vi "Acquire_V2.vi"(5 "Weight Port":refnum<visa-resource-name>, 6 "error in":errorcluster, 7 "GlobalData":T1, 8 "Calibration":variant, 11 "Pressure":refnum<k21>) -> (0 "Weight Port":refnum<visa-resource-name>, 3 "Pressure":refnum<k21>, 4 "error out":errorcluster)   [LabVIEW 2024]
doc: "This the UI responsbile of collection data and display it"
uses:
  controls/GlobalData.ctl
  <vilib>/DAQmx/read.llb/DAQmx Read (Analog 1D DBL NChan 1Samp).vi
  <vilib>/DAQmx/miscellaneous.llb/DAQmx Fill In Error Info.vi
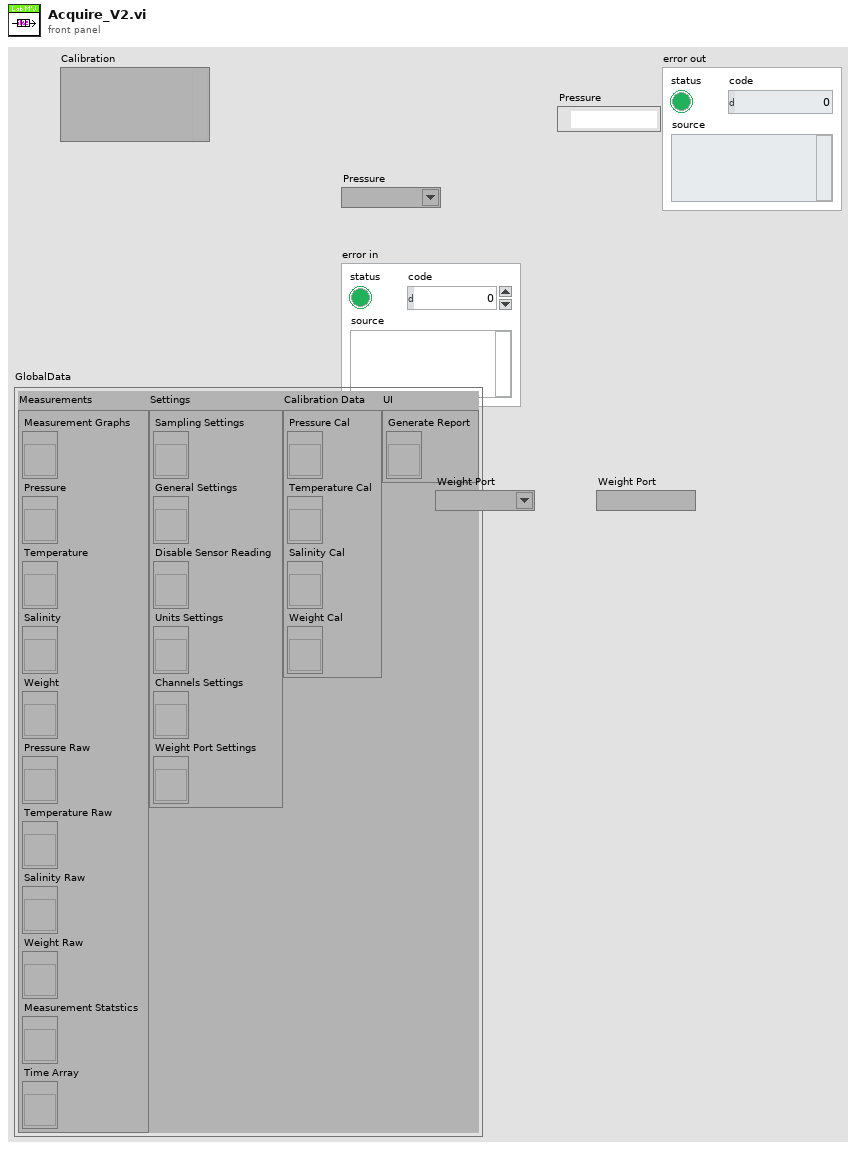
[diagram p1: front panel]
types:
  T1 = typedef "GlobalData.ctl" = cluster{"Measurements":cluster{"Measurement Graphs":refnum<vi>, "Pressure":refnum<vi>, "Temperature":refnum<vi>, "Salinity":refnum<vi>, "Weight":refnum<vi>, "Pressure Raw":refnum<vi>, "Temperature Raw":refnum<vi>, "Salinity Raw":refnum<vi>, "Weight Raw":refnum<vi>, "Measurement Statstics":refnum<vi>, "Time Array":refnum<vi>}, "Settings":cluster{"Sampling Settings":refnum<vi>, "General Settings":refnum<vi>, "Disable Sensor Reading":refnum<vi>, "Units Settings":refnum<vi>, "Channels Settings":refnum<vi>, "Weight Port Settings":refnum<vi>}, "Calibration Data":cluster{"Pressure Cal":refnum<vi>, "Temperature Cal":refnum<vi>, "Salinity Cal":refnum<vi>, "Weight Cal":refnum<vi>}, "UI":cluster{"Generate Report":refnum<vi>}}
  T2 = typedef "Units.ctl" = cluster{"Pressure":enum16{"PSI", "Bar", "atm", "Pa"}, "Temperature":enum16{"C", "K", "F"}, "Salinity":enum16{"ppm", "ppt", "PSU"}, "Weight":enum16{"Kg", "g", "oz", "ib"}}
  T3 = cluster{"C (Y-Intercept)":dbl, "M (Gradient)":dbl}
  T4 = cluster{"Pressure":dbl[], "Temperature":dbl[], "Salinity":dbl[], "Weight":dbl[]}
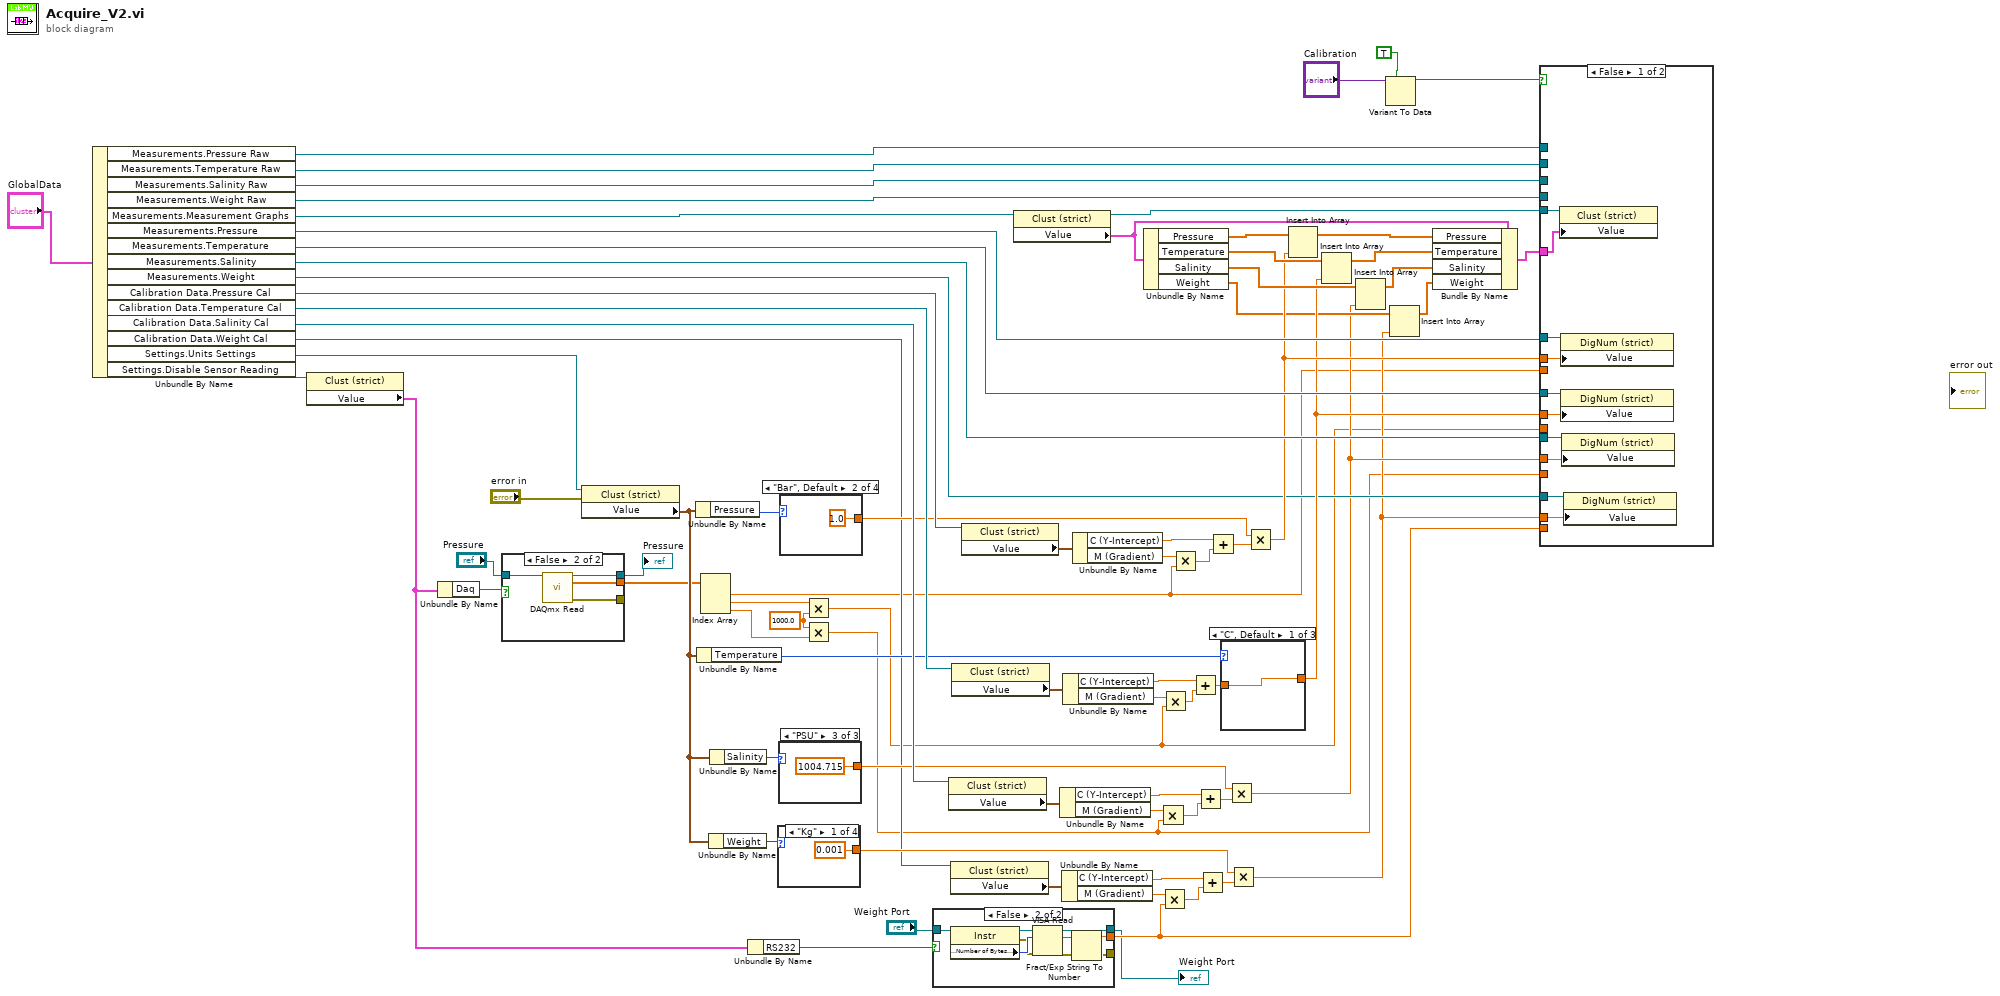
[diagram p0: block diagram]
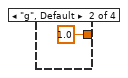
[diagram p2: hidden frame]
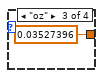
[diagram p3: hidden frame]
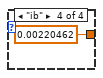
[diagram p4: hidden frame]
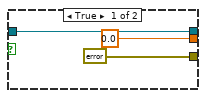
[diagram p5: hidden frame]
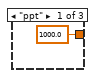
[diagram p6: hidden frame]
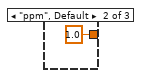
[diagram p7: hidden frame]
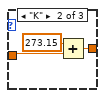
[diagram p8: hidden frame]
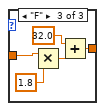
[diagram p9: hidden frame]
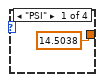
[diagram p10: hidden frame]
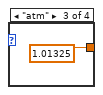
[diagram p11: hidden frame]
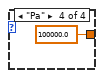
[diagram p12: hidden frame]
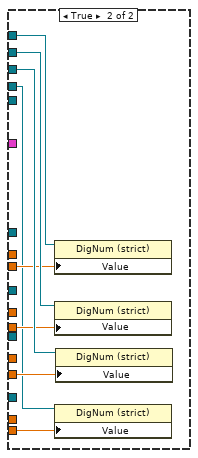
[diagram p13: hidden frame]
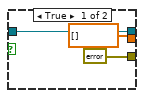
[diagram p14: hidden frame]
diagram:
  w2 = 1000.0 ("C (Y-Intercept)")
  n1 = Unbundle By Name("GlobalData") -> ("Measurements.Pressure Raw"=w49:refnum<vi>, "Measurements.Temperature Raw"=w48:refnum<vi>, "Measurements.Salinity Raw"=w47:refnum<vi>, "Measurements.Weight Raw"=w12:refnum<vi>, "Measurements.Measurement Graphs"=w76:refnum<vi>, "Measurements.Pressure"=w67:refnum<vi>, "Measurements.Temperature"=w66:refnum<vi>, "Measurements.Salinity"=w65:refnum<vi>, "Measurements.Weight"=w26:refnum<vi>, "Calibration Data.Pressure Cal"=w60:refnum<vi>, "Calibration Data.Temperature Cal"=w51:refnum<vi>, "Calibration Data.Salinity Cal"=w50:refnum<vi>, "Calibration Data.Weight Cal"=w17:refnum<vi>, "Settings.Units Settings"=w46:refnum<vi>, "Settings.Disable Sensor Reading"=w10:refnum<vi>)
  n2 = property class="Clust (strict)"(reference=w10) -> ("Value"=w8:cluster{"Daq":bool, "RS232":bool})  [unwired: 1 in, 2 out]
  n3 = Unbundle By Name(w8) -> ("Daq"=w9:bool)
  n4 = case shown="False" w9 {
    tunnel: [w81 w85] -> w78
    tunnel: "Pressure" -> [w81 w84]
    tunnel: [dbl[] [] ("data") w83] -> w6
    tunnel: [errorcluster {"status"=FALSE, "code"=0, "source"=""} ("error out") w82] -> _
    frame True {
    }
    frame False {
      n5 = call-poly <vilib>:"DAQmx Read.vi"("task/channels in"=w84) -> ("task out"=w85:refnum<k21>, "data"=w83:dbl[], "error out"=w82:errorcluster)  [unwired: 12 in]
    }
  }
  "Pressure" <- w78
  n6 = property class="Clust (strict)"(reference=w46, error in="error in") -> ("Value"=w19:T2)  [unwired: 2 out]
  n7 = Unbundle By Name(w19) -> ("Pressure"=w42:enum16{"PSI", "Bar", "atm", "Pa"})
  n8 = Unbundle By Name(w19) -> ("Temperature"=w40:enum16{"C", "K", "F"})
  n9 = Index Array(array=w6) -> (element #1=w11:dbl, element #2=w4:dbl, element #3=w1:dbl)  [unwired: 3 in]
  n10 = Unbundle By Name(w19) -> ("Weight"=w20:enum16{"Kg", "g", "oz", "ib"})
  n11 = Unbundle By Name(w19) -> ("Salinity"=w39:enum16{"ppm", "ppt", "PSU"})
  n12 = Unbundle By Name(w8) -> ("RS232"=w15:bool)
  n13 = case shown="\"Kg\"" w20 {
    tunnel: [0.001 ("C (Y-Intercept)") 1.0 ("C (Y-Intercept)") 0.03527396 ("C (Y-Intercept)") 0.00220462 ("C (Y-Intercept)")] -> w18
    frame "Kg" {
    }
    frame "g", Default {
    }
    frame "oz" {
    }
    frame "ib" {
    }
  }
  n14 = case shown="\"PSU\"" w39 {
    tunnel: [1000.0 ("C (Y-Intercept)") 1.0 ("C (Y-Intercept)") 1004.715 ("C (Y-Intercept)")] -> w38
    frame "ppt" {
    }
    frame "ppm", Default {
    }
    frame "PSU" {
    }
  }
  n15 = case shown="\"Bar\", Default" w42 {
    tunnel: [14.5038 ("C (Y-Intercept)") 1.0 ("C (Y-Intercept)") 1.01325 ("y") 100000.0 ("C (Y-Intercept)")] -> w41
    frame "PSI" {
    }
    frame "Bar", Default {
    }
    frame "atm" {
    }
    frame "Pa" {
    }
  }
  n16 = Multiply(x=w4, y=w2) -> (x*y=w3:dbl)
  n17 = Multiply(x=w2, y=w1) -> (x*y=w5:dbl)
  n18 = case shown="False" w15 {
    tunnel: [w99 w103] -> w7
    tunnel: "Weight Port" -> [w99 w105]
    tunnel: [0.0 ("data") w102] -> w13
    tunnel: [errorcluster {"status"=FALSE, "code"=0, "source"=""} ("error out") w101] -> _
    frame True {
    }
    frame False {
      n19 = property class="Instr"(reference=w105) -> (reference out=w104:refnum<visa-resource-name>, error out=w100:errorcluster, "Serial Settings:Number of Bytes at Serial Port"=w106:u32)  [unwired: 1 in]
      n20 = VISA Read(VISA resource name=w104, byte count=w106, error in (no error)=w100) -> (VISA resource name out=w103:refnum<visa-resource-name>, read buffer=w107:string, error out=w101:errorcluster)  [unwired: 1 out]
      n21 = Fract/Exp String To Number(string=w107) -> (number=w102:dbl)  [unwired: 3 in, 1 out]
    }
  }
  "Weight Port" <- w7
  n22 = property class="Clust (strict)"(reference=w50) -> ("Value"=w55:T3)  [unwired: 1 in, 2 out]
  n23 = property class="Clust (strict)"(reference=w17) -> ("Value"=w21:T3)  [unwired: 1 in, 2 out]
  n24 = property class="Clust (strict)"(reference=w51) -> ("Value"=w56:T3)  [unwired: 1 in, 2 out]
  n25 = property class="Clust (strict)"(reference=w60) -> ("Value"=w64:T3)  [unwired: 1 in, 2 out]
  n26 = property class="Clust (strict)"(reference=w76) -> (reference out=w68:refnum<vi>, "Value"=w73:T4)  [unwired: 1 in, 1 out]
  n27 = Unbundle By Name(w55) -> ("C (Y-Intercept)"=w52:dbl, "M (Gradient)"=w54:dbl)
  n28 = Unbundle By Name(w21) -> ("C (Y-Intercept)"=w24:dbl, "M (Gradient)"=w22:dbl)
  n29 = Unbundle By Name(w56) -> ("C (Y-Intercept)"=w59:dbl, "M (Gradient)"=w57:dbl)
  n30 = Unbundle By Name(w64) -> ("C (Y-Intercept)"=w61:dbl, "M (Gradient)"=w63:dbl)
  n31 = Unbundle By Name(w73) -> ("Pressure"=w75:dbl[], "Temperature"=w71:dbl[], "Salinity"=w70:dbl[], "Weight"=w28:dbl[])
  n32 = Multiply(x=w54, y=w5) -> (x*y=w53:dbl)
  n33 = Multiply(x=w22, y=w13) -> (x*y=w23:dbl)
  n34 = Multiply(x=w57, y=w3) -> (x*y=w58:dbl)
  n35 = Multiply(x=w63, y=w11) -> (x*y=w62:dbl)
  n36 = Add(x=w59, y=w58) -> (x+y=w36:dbl)
  n37 = Add(x=w52, y=w53) -> (x+y=w43:dbl)
  n38 = Add(x=w24, y=w23) -> (x+y=w25:dbl)
  n39 = Add(x=w61, y=w62) -> (x+y=w45:dbl)
  n40 = case shown="\"C\", Default" w40 {
    tunnel: [w108 w111 w116] -> w37
    tunnel: w36 -> [w108 w110 w113]
    frame "C", Default {
    }
    frame "K" {
      n41 = Add(x=273.15, y=w110) -> (x+y=w111:dbl)
    }
    frame "F" {
      n42 = Multiply(x=w113, y=1.8 ("x")) -> (x*y=w114:dbl)
      n43 = Add(x=32.0, y=w114) -> (x+y=w116:dbl)
    }
  }
  n44 = Multiply(x=w38, y=w43) -> (x*y=w16:dbl)
  n45 = Multiply(x=w18, y=w25) -> (x*y=w14:dbl)
  n46 = Multiply(x=w41, y=w45) -> (x*y=w44:dbl)
  n47 = Insert Into Array(array=w75, new element=w44) -> (w74:dbl[])  [unwired: 1 in]
  n48 = Insert Into Array(array=w71, new element=w37) -> (w72:dbl[])  [unwired: 1 in]
  n49 = Insert Into Array(array=w70, new element=w16) -> (w30:dbl[])  [unwired: 1 in]
  n50 = Variant To Data(type=TRUE ("Calibration"), Variant="Calibration") -> (data=w32:bool)  [unwired: 1 in, 1 out]
  n51 = Insert Into Array(array=w28, new element=w14) -> (w29:dbl[])  [unwired: 1 in]
  n52 = Bundle By Name(cluster=w73, "Pressure"=w74, "Temperature"=w72, "Salinity"=w30, "Weight"=w29) -> (w69:T4)
  n53 = case shown="False" w32 {
    tunnel: w69 -> [w126 _]
    tunnel: w68 -> [w125 _]
    tunnel: w67 -> [w124 _]
    tunnel: w66 -> [w123 _]
    tunnel: w65 -> [w122 _]
    tunnel: w44 -> [w121 _]
    tunnel: w37 -> [w120 _]
    tunnel: w16 -> [w119 _]
    tunnel: w49 -> [_ w134]
    tunnel: w48 -> [_ w133]
    tunnel: w47 -> [_ w132]
    tunnel: w11 -> [_ w131]
    tunnel: w3 -> [_ w130]
    tunnel: w5 -> [_ w129]
    tunnel: w26 -> [w118 _]
    tunnel: w14 -> [w117 _]
    tunnel: w13 -> [_ w128]
    tunnel: w12 -> [_ w127]
    frame False {
      n54 = property class="Clust (strict)"(reference=w125, "Value"=w126) -> ()  [unwired: 1 in, 2 out]
      n55 = property class="DigNum (strict)"(reference=w124, "Value"=w121) -> ()  [unwired: 1 in, 2 out]
      n56 = property class="DigNum (strict)"(reference=w123, "Value"=w120) -> ()  [unwired: 1 in, 2 out]
      n57 = property class="DigNum (strict)"(reference=w122, "Value"=w119) -> ()  [unwired: 1 in, 2 out]
      n58 = property class="DigNum (strict)"(reference=w118, "Value"=w117) -> ()  [unwired: 1 in, 2 out]
    }
    frame True {
      n59 = property class="DigNum (strict)"(reference=w134, "Value"=w131) -> ()  [unwired: 1 in, 2 out]
      n60 = property class="DigNum (strict)"(reference=w133, "Value"=w130) -> ()  [unwired: 1 in, 2 out]
      n61 = property class="DigNum (strict)"(reference=w127, "Value"=w128) -> ()  [unwired: 1 in, 2 out]
      n62 = property class="DigNum (strict)"(reference=w132, "Value"=w129) -> ()  [unwired: 1 in, 2 out]
    }
  }
